vi "GetCameraNetworkInfo.vi"(8 "error in (no error)":errorcluster, 10 "network configuration":T1[](array[typedef]) {"IP Address Request Mode" items=["Static"=1, "DHCP/Link Local"=2, "Link-Local Only"=4, "DHCP Only"=8]; "Adapter Mode" items=["Disabled"=1, "TCP/IP Ethernet"=2, "Deterministic"=4, "EtherCAT"=8, "TCP/IP WLAN Connect"=32, "TCP/IP WLAN Create"=64]}, 11 "InterfaceName":string) -> (0 "error out":errorcluster, 1 "local?":bool, 2 "Alias":string, 3 "IPAddress":string)   [LabVIEW 2017]
uses:
  <vilib>/addons/SystemInfoProcess/controls/NetworkAdapterSettings.ctl
  <vilib>/vision/driver/NI_Vision_Acquisition_Software.lvlib
  <resource>/objmgr/imaqdx.rc
  <vilib>/addons/SystemInfoProcess/SystemInfoProcess.lvlib
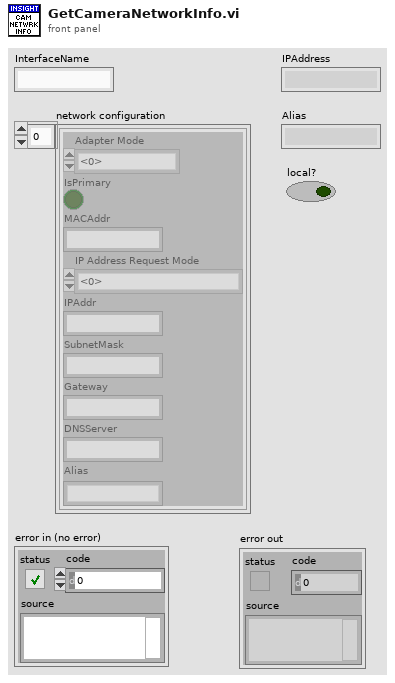
[diagram p1: front panel]
types:
  T1 = typedef "SystemInfoProcess.lvlib/NetworkAdapterSettings.ctl" = cluster{"Adapter Mode":u32, "IsPrimary":bool, "MACAddr":string, "IP Address Request Mode":u32, "IPAddr":string, "SubnetMask":string, "Gateway":string, "DNSServer":string, "Alias":string}
  T2 = typedef "IMAQdx.ctl" = refnum<k21>
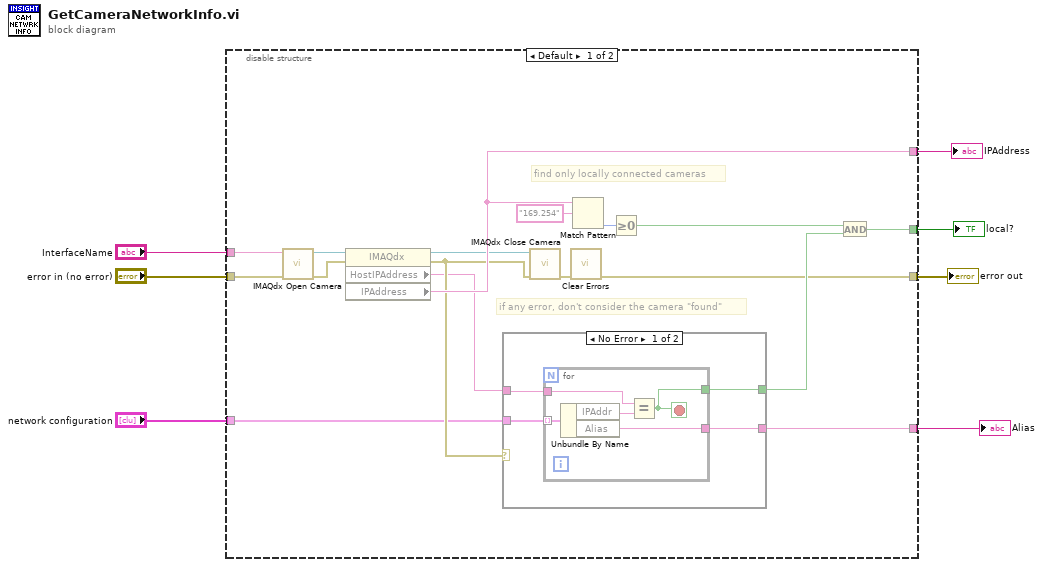
[diagram p0: block diagram]
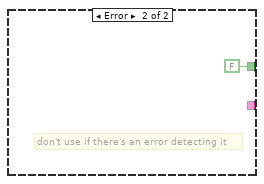
[diagram p2: hidden frame]
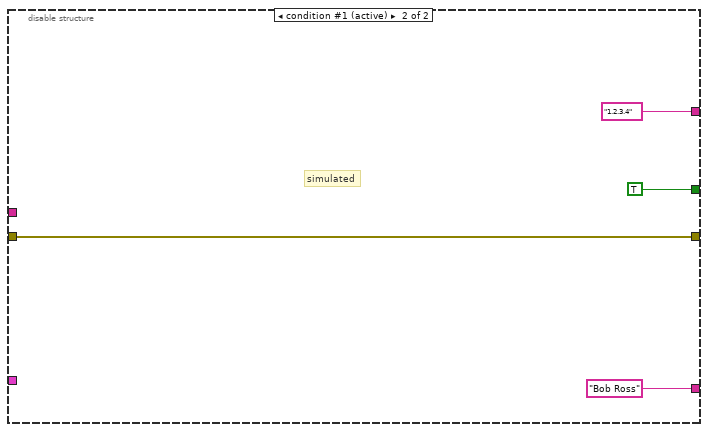
[diagram p3: hidden frame]
diagram:
  n1 = disable-structure shown="Default" {
    disable-tunnel: [w24 TRUE ("local?")] -> w7
    disable-tunnel: [w19 "1.2.3.4" ("IPAddress")] -> w6
    disable-tunnel: [w16 "Bob Ross" ("Alias")] -> w5
    disable-tunnel: "network configuration" -> [w15 _]
    disable-tunnel: "InterfaceName" -> [w13 _]
    disable-tunnel: "error in (no error)" -> [w9 w38]
    disable-tunnel: [w8 w38] -> w1
    frame condition #0 {
      # "if any error, don't consider the camera \"found\""
      # "find only locally connected cameras"
      n2 = call <vilib>:"IMAQdx Open Camera.vi"("error in"=w9, "Session In"=w13) -> ("error out"=w12:errorcluster, "Session Out"=w10:T2)  [unwired: 8 in]
      n3 = property class="IMAQdx"(reference=w10, error in=w12) -> (reference out=w11:T2, error out=w17:errorcluster, "HostIPAddress"=w14:string, "IPAddress"=w19:string)
      n4 = case shown="No Error" w17 {
        tunnel: w14 -> [w28 _]
        tunnel: w15 -> [w27 _]
        tunnel: [w26 _] -> w16
        tunnel: [w25 FALSE] -> w23
        frame No Error {
          n5 = for {
            tunnel: w28 -> [w31]
            tunnel: w27 -> [w33] mode=indexing
            tunnel: [w30] -> w26
            tunnel: [w29] -> w25
            stop <- w29 stop-if-true
            n6 = Unbundle By Name(w33) -> ("IPAddr"=w32:string, "Alias"=w30:string)
            n7 = Equal?(x=w31, y=w32) -> (x = y?=w29:bool)
          }
        }
        frame Error {
          # "don't use if there's an error detecting it"
        }
      }
      n8 = call <vilib>:"IMAQdx Close Camera.vi"("error in"=w17, "Session In"=w11) -> ("error out"=w18:errorcluster)  [unwired: 9 in]
      n9 = call <vilib>:"Clear Errors.vi"("error in (no error)"=w18) -> ("error out"=w8:errorcluster)  [unwired: 5 in, 1 out]
      n10 = Match Pattern(string=w19, regular expression="169.254") -> (offset past match=w21:i32)  [unwired: 1 in, 3 out]
      n11 = Greater Or Equal To 0?(x=w21) -> (x >= 0?=w22:bool)
      n12 = And(x=w22, y=w23) -> (x .and. y?=w24:bool)
    }
    frame condition #1 (active) {
      # "simulated"
    }
  }
  "local?" <- w7
  "IPAddress" <- w6
  "Alias" <- w5
  "error out" <- w1
